vi "5_9.vi"() -> ()   [LabVIEW 2015]
panel:
  out "C":dbl
  in  "B":dbl
  in  "A":dbl
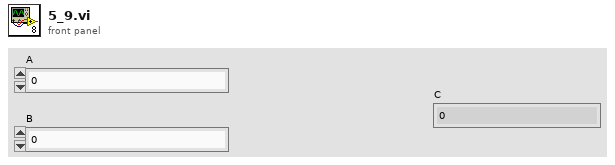
[diagram p1: front panel]
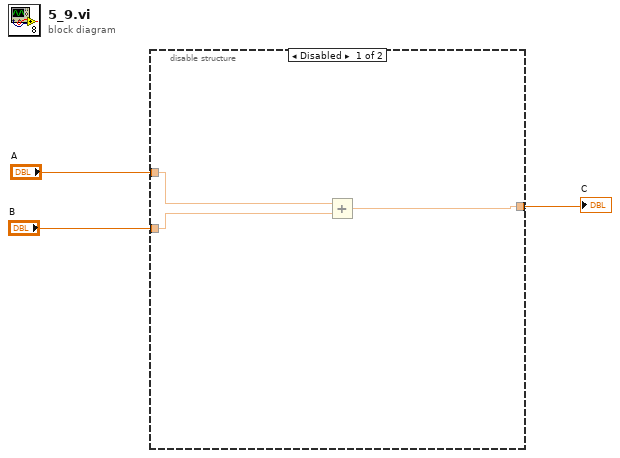
[diagram p0: block diagram]
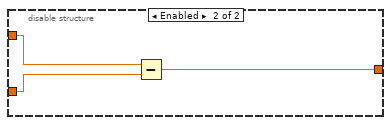
[diagram p2: hidden frame]
diagram:
  n1 = disable-structure shown="Disabled" {
    disable-tunnel: "A" -> [w6 w9]
    disable-tunnel: "B" -> [w5 w8]
    disable-tunnel: [w4 w7] -> w1
    frame Disabled {
      n2 = Add(x=w6, y=w5) -> (x+y=w4:dbl)
    }
    frame Enabled {
      n3 = Subtract(x=w9, y=w8) -> (x-y=w7:dbl)
    }
  }
  "C" <- w1
